vi "LogColumnData.vi"(8 "Error In":errorcluster, 11 "MasterCluster In":T1={"Plate Reader State"=enum."Idle", "SMPAutomationClientRef"=refnum, "CommandCompleted Refnum"=refnum, "InstrumentStatusChanged Refnum"=refnum, "ErrorReport Refnum"=refnum, "Read Start Time"=timestamp(0 s since 1904-01-01), "Read Count"=0, "Active Column"=0, "Raw Result"="", "GetDataCopy CMD Queue ID"=0, "Error Log"="", "Column Data"={"Col Absorbances"=[], "Col Read Times"=[], "Col Read Positions (deg)"=[], "Temperature (degC)"=0.0, "Active Column"=0, "Previous Column"=0, "Column Read Start Time"=timestamp(0 s since 1904-01-01), "Column Busy Start Time"=timestamp(0 s since 1904-01-01), "Column Busy Stop Time"=timestamp(0 s since 1904-01-01), "Column Mark Read Start Time"=timestamp(0 s since 1904-01-01), "Column Mark Read Stop Time"=timestamp(0 s since 1904-01-01)}, "Grid"=[[0.0, 0.0, 0.0, 0.0, 0.0, 0.0, 0.0, 0.0, 0.0, 0.0, 0.0, 0.0], [0.0, 0.0, 0.0, 0.0, 0.0, 0.0, 0.0, 0.0, 0.0, 0.0, 0.0, 0.0], [0.0, 0.0, 0.0, 0.0, 0.0, 0.0, 0.0, 0.0, 0.0, 0.0, 0.0, 0.0], [0.0, 0.0, 0.0, 0.0, 0.0, 0.0, 0.0, 0.0, 0.0, 0.0, 0.0, 0.0], [0.0, 0.0, 0.0, 0.0, 0.0, 0.0, 0.0, 0.0, 0.0, 0.0, 0.0, 0.0], [0.0, 0.0, 0.0, 0.0, 0.0, 0.0, 0.0, 0.0, 0.0, 0.0, 0.0, 0.0], [0.0, 0.0, 0.0, 0.0, 0.0, 0.0, 0.0, 0.0, 0.0, 0.0, 0.0, 0.0], [0.0, 0.0, 0.0, 0.0, 0.0, 0.0, 0.0, 0.0, 0.0, 0.0, 0.0, 0.0]], "Column Read Start Time"=timestamp(0 s since 1904-01-01), "Previous Column"=0, "Raw Log File Refnum"=refnum, "Read Specifications"={"Read Period (min)"=0.0, "Experiment Duration (min)"=0.0, "Number of Columns"=0, "Apex Deviance (deg)"=0.0, "Log File Name"="", "Number of Wavelengths"=0, "Timing Profile"=enum."No Timing", "Column Switch Delay"=0.0, "Column Repeat Delay"=0.0, "Audible Read Delay"=0.0, "Audible Read Interval"=0.0, "SMP Protocol Path"=path "", "Upper Busy Delay Limit"=inf, "Lower Busy Delay Limit"=-inf, "Upper Busy Interval Limit"=inf, "Lower Busy Interval Limit"=-inf, "Number of Rows"=0, "Plate Reader COM Port"=""}, "Plate Reader Crash State"=enum."Idle", "Consecutive Missed Reads"=0, "Excel File Refnum"=refnum} {"Column Data"."Column Mark Read Stop Time" format="%<%H:%M:%S%3u\n%x>T"; "Column Data"."Column Mark Read Start Time" format="%<%H:%M:%S%3u\n%x>T"; "Column Data"."Column Busy Stop Time" format="%<%H:%M:%S%3u\n%x>T"; "Column Data"."Column Busy Start Time" format="%<%H:%M:%S%3u\n%x>T"; "Column Data"."Column Read Start Time" format="%<%H:%M:%S%3u\n%x>T"; "Column Data"."Col Read Times" format="%<%H:%M:%S%3u\n%x>T"}) -> (0 "Error Out":errorcluster, 3 "MasterCluster Out":T1={"Plate Reader State"=enum."Idle", "SMPAutomationClientRef"=refnum, "CommandCompleted Refnum"=refnum, "InstrumentStatusChanged Refnum"=refnum, "ErrorReport Refnum"=refnum, "Read Start Time"=timestamp(0 s since 1904-01-01), "Read Count"=0, "Active Column"=0, "Raw Result"="", "GetDataCopy CMD Queue ID"=0, "Error Log"="", "Column Data"={"Col Absorbances"=[], "Col Read Times"=[], "Col Read Positions (deg)"=[], "Temperature (degC)"=0.0, "Active Column"=0, "Previous Column"=0, "Column Read Start Time"=timestamp(0 s since 1904-01-01), "Column Busy Start Time"=timestamp(0 s since 1904-01-01), "Column Busy Stop Time"=timestamp(0 s since 1904-01-01), "Column Mark Read Start Time"=timestamp(0 s since 1904-01-01), "Column Mark Read Stop Time"=timestamp(0 s since 1904-01-01)}, "Grid"=[[0.0, 0.0, 0.0, 0.0, 0.0, 0.0, 0.0, 0.0, 0.0, 0.0, 0.0, 0.0], [0.0, 0.0, 0.0, 0.0, 0.0, 0.0, 0.0, 0.0, 0.0, 0.0, 0.0, 0.0], [0.0, 0.0, 0.0, 0.0, 0.0, 0.0, 0.0, 0.0, 0.0, 0.0, 0.0, 0.0], [0.0, 0.0, 0.0, 0.0, 0.0, 0.0, 0.0, 0.0, 0.0, 0.0, 0.0, 0.0], [0.0, 0.0, 0.0, 0.0, 0.0, 0.0, 0.0, 0.0, 0.0, 0.0, 0.0, 0.0], [0.0, 0.0, 0.0, 0.0, 0.0, 0.0, 0.0, 0.0, 0.0, 0.0, 0.0, 0.0], [0.0, 0.0, 0.0, 0.0, 0.0, 0.0, 0.0, 0.0, 0.0, 0.0, 0.0, 0.0], [0.0, 0.0, 0.0, 0.0, 0.0, 0.0, 0.0, 0.0, 0.0, 0.0, 0.0, 0.0]], "Column Read Start Time"=timestamp(0 s since 1904-01-01), "Previous Column"=0, "Raw Log File Refnum"=refnum, "Read Specifications"={"Read Period (min)"=0.0, "Experiment Duration (min)"=0.0, "Number of Columns"=0, "Apex Deviance (deg)"=0.0, "Log File Name"="", "Number of Wavelengths"=0, "Timing Profile"=enum."No Timing", "Column Switch Delay"=0.0, "Column Repeat Delay"=0.0, "Audible Read Delay"=0.0, "Audible Read Interval"=0.0, "SMP Protocol Path"=path "", "Upper Busy Delay Limit"=inf, "Lower Busy Delay Limit"=-inf, "Upper Busy Interval Limit"=inf, "Lower Busy Interval Limit"=-inf, "Number of Rows"=0, "Plate Reader COM Port"=""}, "Plate Reader Crash State"=enum."Idle", "Consecutive Missed Reads"=0, "Excel File Refnum"=refnum} {"Column Data"."Column Mark Read Stop Time" format="%<%H:%M:%S%3u\n%x>T"; "Column Data"."Column Mark Read Start Time" format="%<%H:%M:%S%3u\n%x>T"; "Column Data"."Column Busy Stop Time" format="%<%H:%M:%S%3u\n%x>T"; "Column Data"."Column Busy Start Time" format="%<%H:%M:%S%3u\n%x>T"; "Column Data"."Column Read Start Time" format="%<%H:%M:%S%3u\n%x>T"; "Column Data"."Col Read Times" format="%<%H:%M:%S%3u\n%x>T"})   [LabVIEW 2014]
uses:
  MasterCluster.ctl
  PlateReaderState.ctl
  C:/Program Files (x86)/Molecular Devices/SoftMax Pro 6.5.1 Automation SDK/SoftMaxPro.AutomationClient.dll
  Program Files (x86)/Molecular Devices/SoftMax Pro 6.5.1 Automation SDK/SoftMaxPro.AutomationClient.dll
  ColumnData.ctl
  ReadSpecifications.ctl
  TimingProfile.ctl
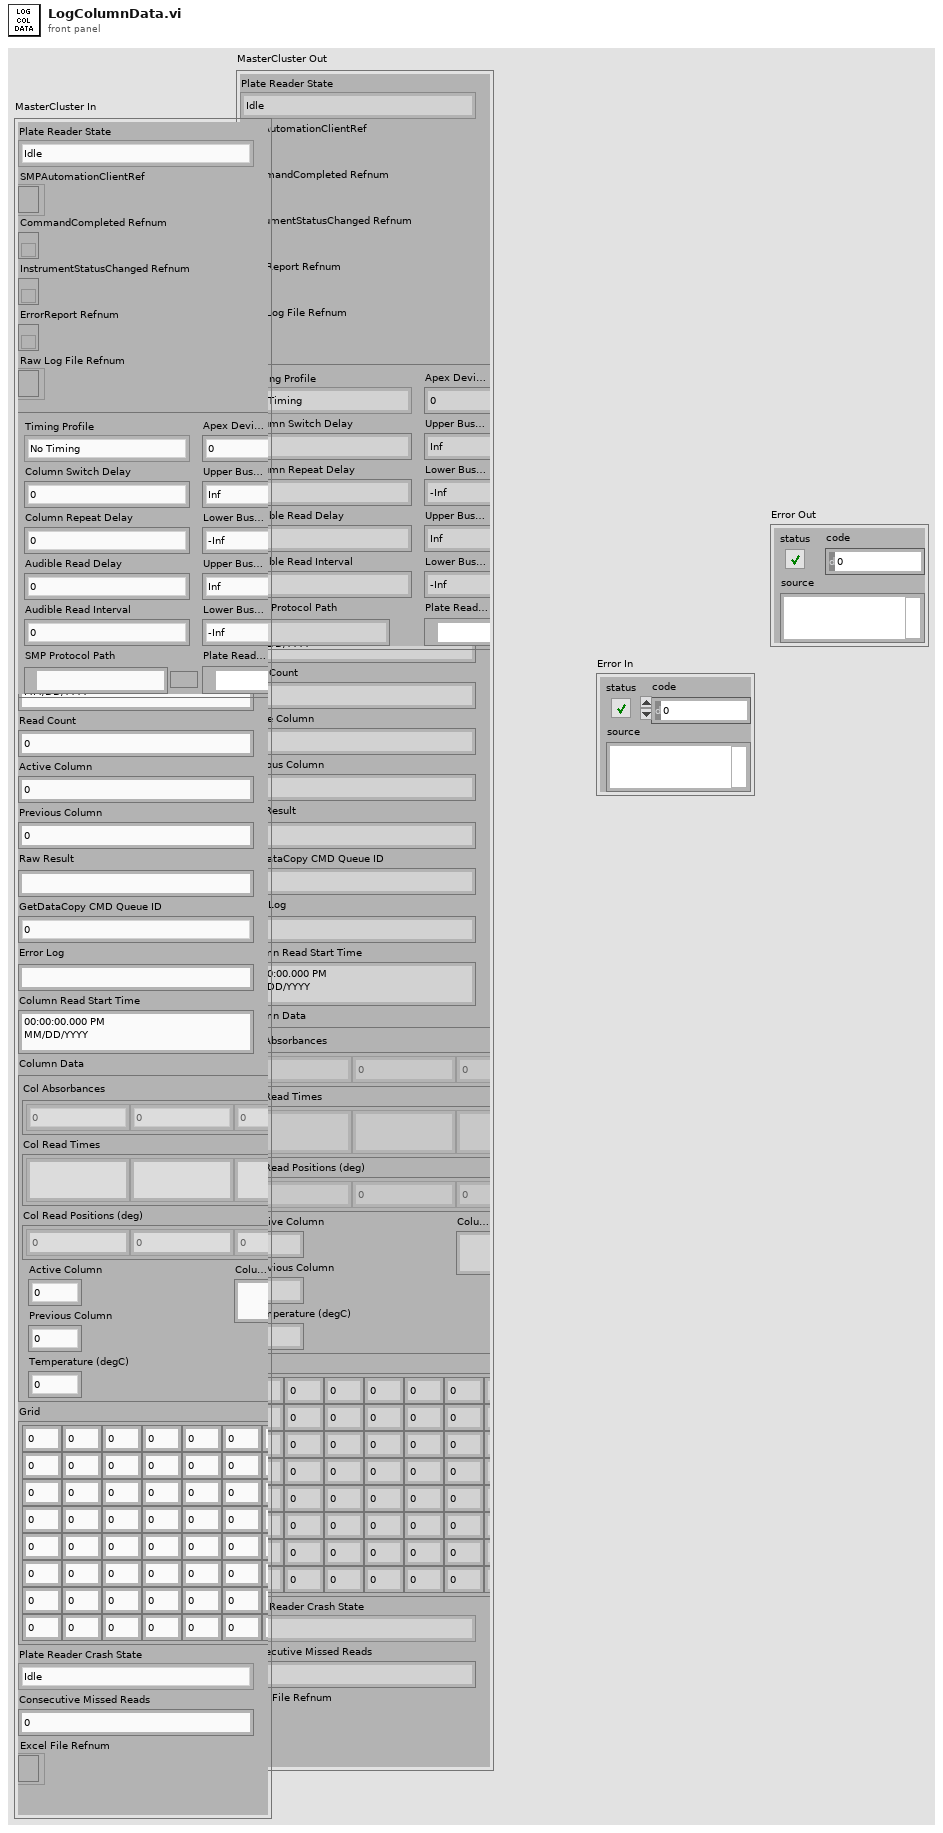
[diagram p1: front panel]
types:
  T1 = typedef "MasterCluster.ctl" = cluster{"Plate Reader State":T2, "SMPAutomationClientRef":refnum<k24>, "CommandCompleted Refnum":refnum<k27>, "InstrumentStatusChanged Refnum":refnum<k27>, "ErrorReport Refnum":refnum<k27>, "Read Start Time":timestamp, "Read Count":u64, "Active Column":u64, "Raw Result":string, "GetDataCopy CMD Queue ID":i32, "Error Log":string, "Column Data":T3, "Grid":dbl[][], "Column Read Start Time":timestamp, "Previous Column":u64, "Raw Log File Refnum":refnum<file>, "Read Specifications":T4, "Plate Reader Crash State":T2, "Consecutive Missed Reads":u64, "Excel File Refnum":refnum<file>}
  T2 = typedef "PlateReaderState.ctl" = enum16{"Idle", "Run", "Wait", "Read", "Init", "Exit", "Stop"}
  T3 = typedef "ColumnData.ctl" = cluster{"Col Absorbances":dbl[], "Col Read Times":timestamp[], "Col Read Positions (deg)":dbl[], "Temperature (degC)":dbl, "Active Column":u64, "Previous Column":u64, "Column Read Start Time":timestamp, "Column Busy Start Time":timestamp, "Column Busy Stop Time":timestamp, "Column Mark Read Start Time":timestamp, "Column Mark Read Stop Time":timestamp}
  T4 = typedef "ReadSpecifications.ctl" = cluster{"Read Period (min)":dbl, "Experiment Duration (min)":dbl, "Number of Columns":u64, "Apex Deviance (deg)":dbl, "Log File Name":string, "Number of Wavelengths":u64, "Timing Profile":T5, "Column Switch Delay":dbl, "Column Repeat Delay":dbl, "Audible Read Delay":dbl, "Audible Read Interval":dbl, "SMP Protocol Path":path, "Upper Busy Delay Limit":dbl, "Lower Busy Delay Limit":dbl, "Upper Busy Interval Limit":dbl, "Lower Busy Interval Limit":dbl, "Number of Rows":u64, "Plate Reader COM Port":refnum<visa-resource-name>}
  T5 = typedef "TimingProfile.ctl" = enum16{"No Timing", "24-Well Fluorescence", "48-Well Fluorescence", "96-Well Fluorescence", "96-Well Absorbance", "Custom Timing"}
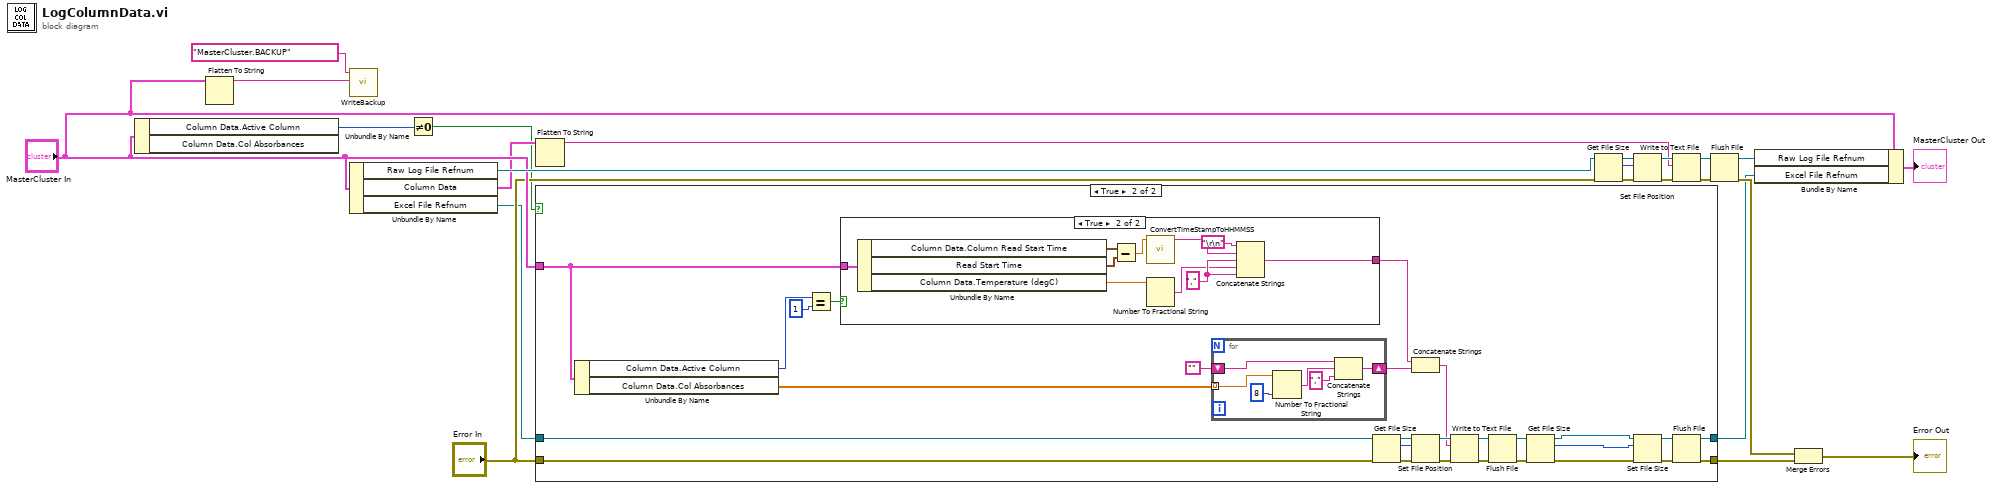
[diagram p0: block diagram]
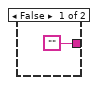
[diagram p3: hidden frame]
diagram:
  n1 = Unbundle By Name("MasterCluster In") -> ("Column Data.Active Column"=w2:u64)  [unwired: 1 out]
  n2 = Flatten To String(anything="MasterCluster In") -> (data string=w11:string)  [unwired: 3 in, 2 out]
  n3 = call "WriteBackup.vi"("Backup Data"=w11, "Backup Name"="MasterCluster.BACKUP" ("name or relative path")) -> ()  [unwired: 10 in]
  n4 = Unbundle By Name("MasterCluster In") -> ("Raw Log File Refnum"=w18:refnum<file>, "Column Data"=w5:T3, "Excel File Refnum"=w6:refnum<file>)
  n5 = Not Equal To 0?(x=w2) -> (x != 0?=w1:bool)
  n6 = Flatten To String(anything=w5) -> (data string=w15:string)  [unwired: 3 in, 2 out]
  n7 = case shown="True" w1 {
    tunnel: "MasterCluster In" -> [_ w31]
    tunnel: "Error In" -> [w24 w48]
    tunnel: w6 -> [w25 w42]
    tunnel: [w24 w41] -> w4
    tunnel: [w25 w40] -> w3
    frame False {
    }
    frame True {
      n8 = Unbundle By Name(w31) -> ("Column Data.Active Column"=w28:u64, "Column Data.Col Absorbances"=w30:dbl[])
      n9 = Equal?(x=w28, y=u64 1) -> (x = y?=w27:bool)
      n10 = case shown="True" w27 {
        tunnel: w31 -> [_ w69]
        tunnel: ["" w61] -> w52
        frame False {
        }
        frame True {
          w65 = "," ("string")
          n11 = Unbundle By Name(w69) -> ("Column Data.Column Read Start Time"=w68:timestamp, "Read Start Time"=w67:timestamp, "Column Data.Temperature (degC)"=w66:dbl)
          n12 = Subtract(x=w68, y=w67) -> (x-y=w64:dbl)
          n13 = call "ConvertTimeStampToHHMMSS.vi"("Timestamp"=w64) -> ("HH:MM:SS"=w63:string)  [unwired: 10 in]
          n14 = Number To Fractional String(number=w66) -> (F-format string=w62:string)  [unwired: 3 in]
          n15 = Concatenate Strings("\r\n", w63, w65, w62, w65) -> (w61:string)
        }
      }
      n16 = for {
        tunnel: w30 -> [w58] mode=indexing
        shift-right: [w55] -> w50
        shift-left: "" -> [w56]
        n17 = Number To Fractional String(number=w58, precision (6)=i16 8) -> (F-format string=w54:string)  [unwired: 2 in]
        n18 = Concatenate Strings(w56, w54, "," ("string")) -> (w55:string)
      }
      n19 = Get File Size(file=w42, error in=w48) -> (refnum out=w47:refnum<file>, size (in bytes)=w46:i64, 0:w49:errorcluster)
      n20 = Concatenate Strings(w52, w50) -> (w43:string)
      n21 = Set File Position(offset (in bytes) (0)=w46, refnum=w47, error in=w49) -> (refnum out=w44:refnum<file>, error out=w45:errorcluster)  [unwired: 1 in]
      n22 = Write to Text File(file (use dialog)=w44, text=w43, error in=w45) -> (refnum out=w35:refnum<file>, error out=w34:errorcluster)  [unwired: 1 in, 1 out]
      n23 = Flush File(refnum=w35, error in=w34) -> (refnum out=w32:refnum<file>, error out=w33:errorcluster)
      n24 = Get File Size(file=w32, error in=w33) -> (refnum out=w39:refnum<file>, size (in bytes)=w26:i64, 0:w38:errorcluster)
      n25 = Set File Size(4:w38, 6:w26, 7:w39) -> (0:w36:errorcluster, 3:w37:refnum<file>)
      n26 = Flush File(refnum=w37, error in=w36) -> (refnum out=w40:refnum<file>, error out=w41:errorcluster)
    }
  }
  n27 = Get File Size(file=w18, error in="Error In") -> (refnum out=w22:refnum<file>, size (in bytes)=w21:i64, 0:w23:errorcluster)
  n28 = Set File Position(offset (in bytes) (0)=w21, refnum=w22, error in=w23) -> (refnum out=w20:refnum<file>, error out=w19:errorcluster)  [unwired: 1 in]
  n29 = Write to Text File(file (use dialog)=w20, text=w15, error in=w19) -> (refnum out=w14:refnum<file>, error out=w13:errorcluster)  [unwired: 1 in, 1 out]
  n30 = Flush File(refnum=w14, error in=w13) -> (refnum out=w16:refnum<file>, error out=w7:errorcluster)
  n31 = Bundle By Name(cluster="MasterCluster In", "Raw Log File Refnum"=w16, "Excel File Refnum"=w3) -> (→"MasterCluster Out":T1)
  n32 = Merge Errors(w7, w4) -> (→"Error Out":errorcluster)
